vi "XY plotter follower program.vi"() -> ()   [LabVIEW 2019]
panel:
  out "Homed?":bool
  out "Ready?":bool
  out "y":dbl
  out "x":dbl
  in  "stop":bool
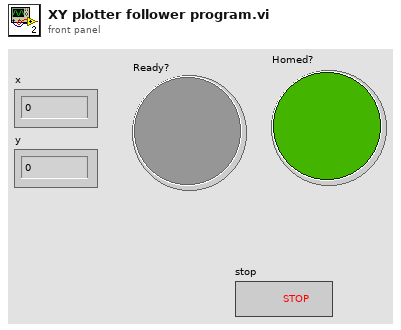
[diagram p1: front panel]
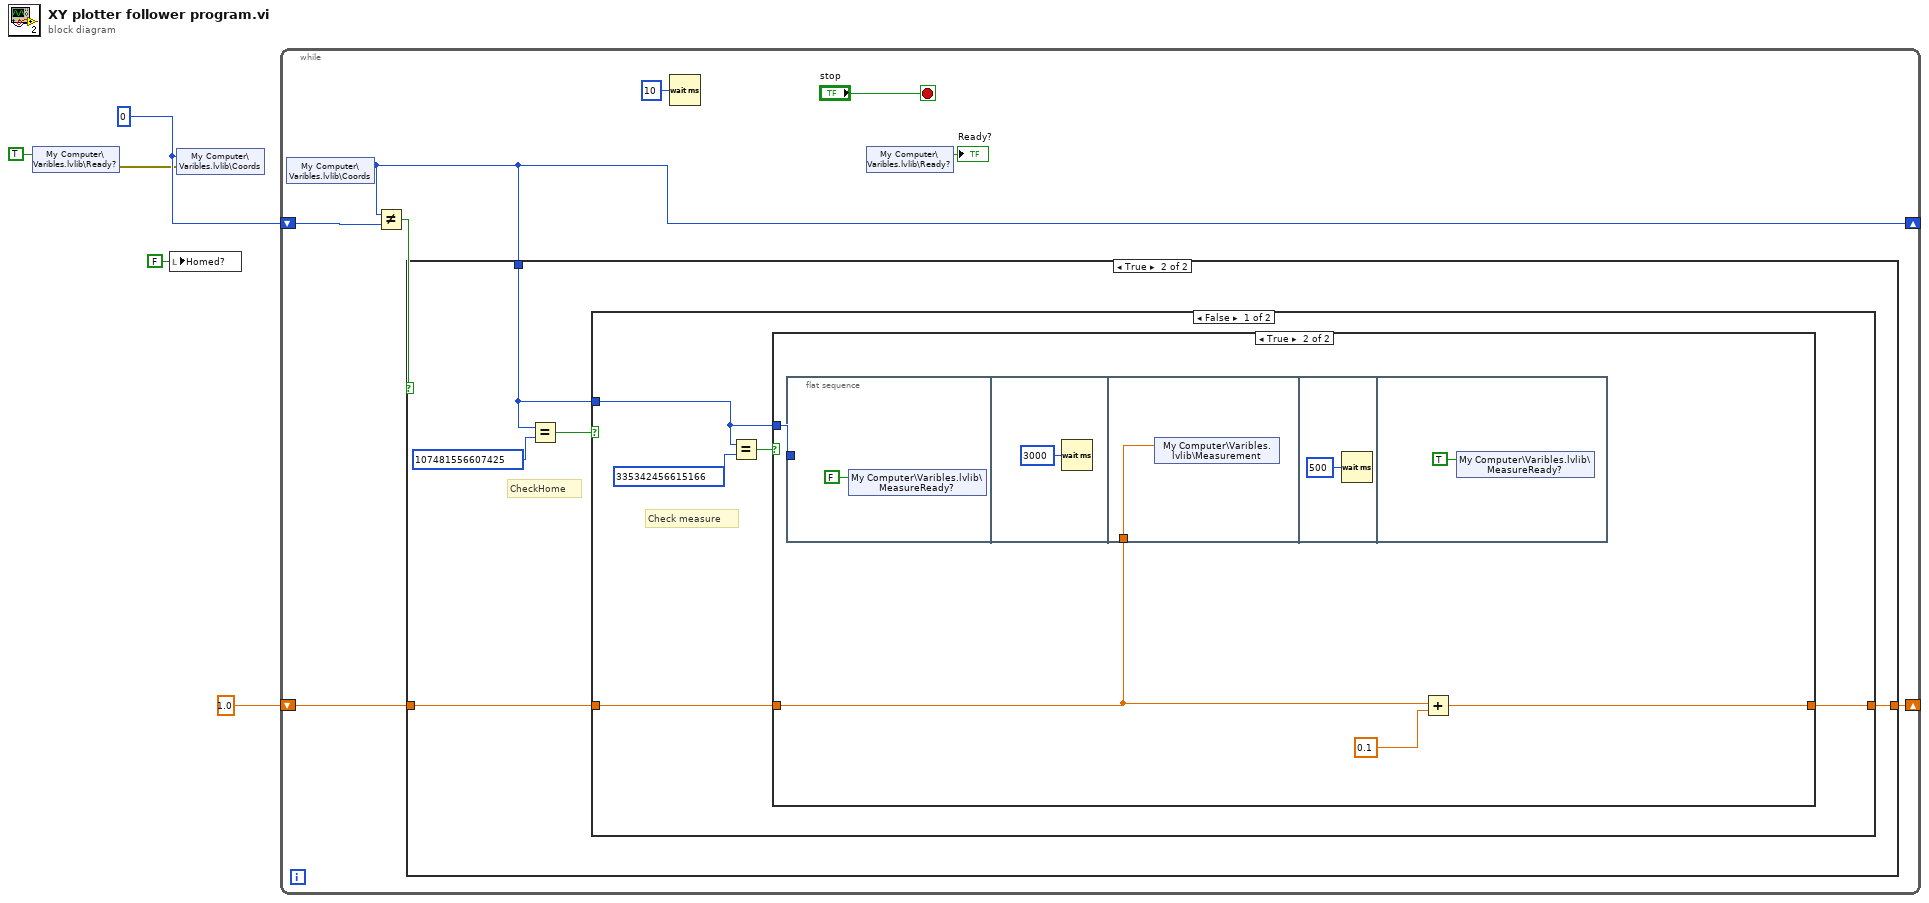
[diagram p0: block diagram]
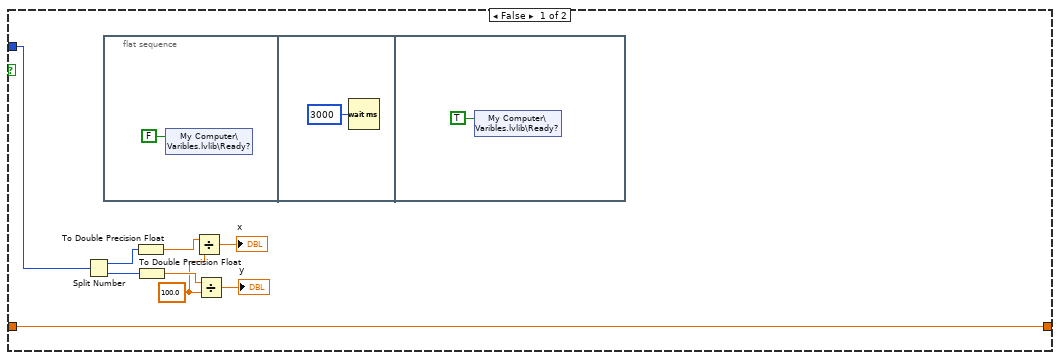
[diagram p3: hidden frame]
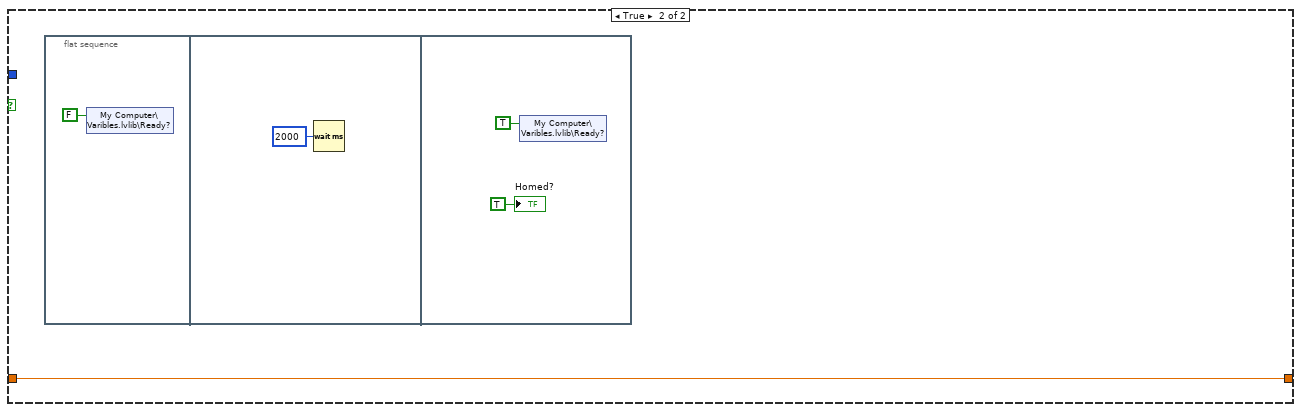
[diagram p4: hidden frame]
diagram:
  w5 = u64 0 ("Coords")
  n1 = shared-variable "My Computer\\Varibles.lvlib\\Ready?"(TRUE ("Ready?")) -> (error out=w3:errorcluster)  [unwired: 1 in]
  n2 = local write "Homed?"(FALSE ("Homed?")) -> ()
  n3 = shared-variable "My Computer\\Varibles.lvlib\\Coords"(w5, error in=w3) -> ()  [unwired: 1 out]
  n4 = while {
    shift-right: [w9] -> _
    shift-left: w5 -> [w11]
    shift-right: [w7] -> _
    shift-left: 1.0 -> [w8]
    stop <- "stop" stop-if-true
    n5 = shared-variable "My Computer\\Varibles.lvlib\\Coords"() -> (w9:u64)  [unwired: 1 in, 1 out]
    n6 = Not Equal?(x=w9, y=w11) -> (x != y?=w10:bool)
    n7 = case shown="True" w10 {
      tunnel: w9 -> [_ w15]
      tunnel: w8 -> [w14 w17]
      tunnel: [w14 w16] -> w7
      frame False {
      }
      frame True {
        # "CheckHome"
        n8 = Equal?(x=w15, y=u64 107481556607425) -> (x = y?=w18:bool)
        n9 = case shown="False" w18 {
          tunnel: w17 -> [w21 w46]
          tunnel: [w20 w46] -> w16
          tunnel: w15 -> [w22 _]
          frame False {
            # "Check measure"
            n10 = Equal?(x=w22, y=u64 335342456615166) -> (x = y?=w23:bool)
            n11 = case shown="True" w23 {
              tunnel: w22 -> [w25 w40]
              tunnel: w21 -> [w33 w39]
              tunnel: [w33 w38] -> w20
              frame False {
                w26 = 100.0 ("y")
                n12 = Split Number(x=w25) -> (hi(x)=w32:u32, lo(x)=w31:u32)
                n13 = flat-sequence {
                  frame #0 {
                    n14 = shared-variable "My Computer\\Varibles.lvlib\\Ready?"(FALSE ("Ready?")) -> ()  [unwired: 1 in, 1 out]
                  }
                  frame #1 {
                    n15 = Wait (ms)(milliseconds to wait=u32 3000) -> ()  [unwired: 1 out]
                  }
                  frame #2 {
                    n16 = shared-variable "My Computer\\Varibles.lvlib\\Ready?"(TRUE ("Ready?")) -> ()  [unwired: 1 in, 1 out]
                  }
                }
                n17 = To Double Precision Float(number=w32) -> (double precision float=w30:dbl)
                n18 = To Double Precision Float(number=w31) -> (double precision float=w29:dbl)
                n19 = Divide(x=w30, y=w26) -> (x/y=→"x":dbl)
                n20 = Divide(x=w29, y=w26) -> (x/y=→"y":dbl)
              }
              frame True {
                n21 = flat-sequence {
                  tunnel: w40 -> [_]
                  tunnel: w39 -> [w43]
                  frame #0 {
                    n22 = shared-variable "My Computer\\Varibles.lvlib\\MeasureReady?"(FALSE ("Ready?")) -> ()  [unwired: 1 in, 1 out]
                  }
                  frame #1 {
                    n23 = Wait (ms)(milliseconds to wait=u32 3000) -> ()  [unwired: 1 out]
                  }
                  frame #2 {
                    n24 = shared-variable "My Computer\\Varibles.lvlib\\Measurement"(w43) -> ()  [unwired: 1 in, 1 out]
                  }
                  frame #3 {
                    n25 = Wait (ms)(milliseconds to wait=u32 500) -> ()  [unwired: 1 out]
                  }
                  frame #4 {
                    n26 = shared-variable "My Computer\\Varibles.lvlib\\MeasureReady?"(TRUE ("Ready?")) -> ()  [unwired: 1 in, 1 out]
                  }
                }
                n27 = Add(x=w39, y=0.1 ("x")) -> (x+y=w38:dbl)
              }
            }
          }
          frame True {
            n28 = flat-sequence {
              frame #0 {
                n29 = shared-variable "My Computer\\Varibles.lvlib\\Ready?"(FALSE ("Ready?")) -> ()  [unwired: 1 in, 1 out]
              }
              frame #1 {
                n30 = Wait (ms)(milliseconds to wait=u32 2000) -> ()  [unwired: 1 out]
              }
              frame #2 {
                n31 = shared-variable "My Computer\\Varibles.lvlib\\Ready?"(TRUE ("Ready?")) -> ()  [unwired: 1 in, 1 out]
                "Homed?" <- TRUE ("Homed?")
              }
            }
          }
        }
      }
    }
    n32 = Wait (ms)(milliseconds to wait=u32 10) -> ()  [unwired: 1 out]
    n33 = shared-variable "My Computer\\Varibles.lvlib\\Ready?"() -> (→"Ready?":bool)  [unwired: 1 in, 1 out]
  }
